vi "Write Attributes.vi"(8 "error in (no error)":errorcluster, 10 "Attributes":refnum<class "Attribute.lvclass">[](array[class]), 11 "Element in":refnum<class "Element.lvclass">) -> (0 "error out":errorcluster, 3 "Element out":refnum<class "Element.lvclass">)   [LabVIEW 2026]
uses:
  Element.lvclass
  Attribute/Attribute.lvclass
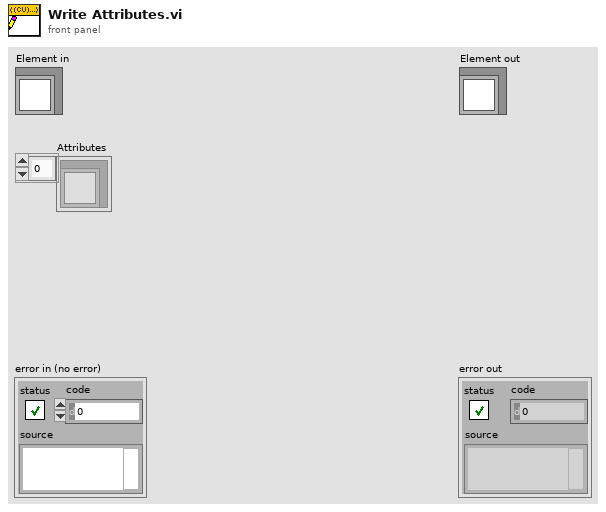
[diagram p1: front panel]
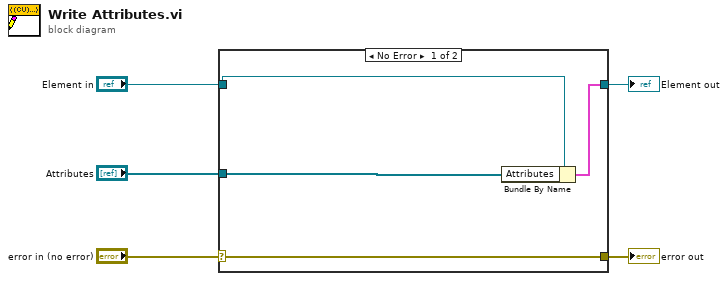
[diagram p0: block diagram]
diagram:
  n1 = case shown="No Error" "error in (no error)" {
    selector: "error in (no error)" -> [w9 w10]
    tunnel: [w9 w10] -> w4
    tunnel: [w7 w11] -> w2
    tunnel: "Element in" -> [w8 w11]
    tunnel: "Attributes" -> [w6 _]
    frame No Error {
      n2 = Bundle By Name(cluster=w8, "Attributes"=w6) -> (w7:cluster{})
    }
    frame Error {
    }
  }
  "error out" <- w4
  "Element out" <- w2
